vi "Get List Information.vi"(7 "App Instance":refnum<vi>, 8 "Tree DQMH Sel":string, 9 "DQMH Scan Info":T2, 11 "Tree Map":T4) -> (1 "Broadcast?":bool, 2 "Vi out":refnum<vi>, 3 "Module type":T1, 5 "DQMH Lib":refnum<vi>)   [LabVIEW 2019, in "Panther Dashboard.lvlib"]
uses:
  Panther Dashboard.lvlib
  <vilib>/National Instruments/Tree Map/Tree Map Data.ctl
  DQMH Modules Info--cluster.ctl
  Module type--enum.ctl
  Project References--cluster.ctl
  <vilib>/National Instruments/Tree Map/Tree Map.lvlib
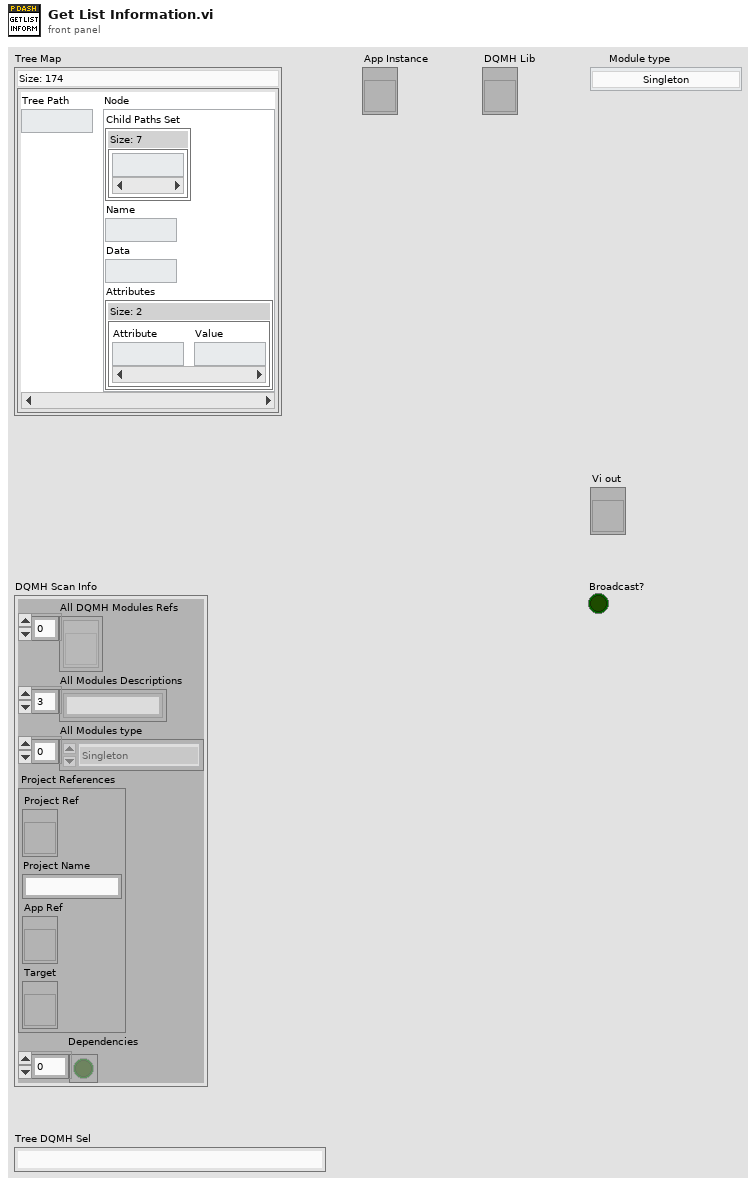
[diagram p1: front panel]
types:
  T1 = typedef "Panther Dashboard.lvlib/Module type--enum.ctl" = enum16{"Singleton", "Cloneable"}
  T2 = typedef "Panther Dashboard.lvlib/DQMH Modules Info--cluster.ctl" = cluster{"All DQMH Modules Refs":refnum<vi>[], "All Modules Descriptions":string[], "All Modules type":T1[], "Project References":T3, "Dependencies":bool[]}
  T3 = typedef "Panther Dashboard.lvlib/Project References--cluster.ctl" = cluster{"Project Ref":refnum<vi>, "Project Name":string, "App Ref":refnum<vi>, "Target":refnum<vi>}
  T4 = typedef "Tree Map.lvlib/Tree Map Data.ctl" = map{string, cluster{"Child Paths Set":set{string}, "Name":string, "Data":string, "Attributes":map{string, string}}}
  T5 = cluster{"Description":string, "VI Description":string}
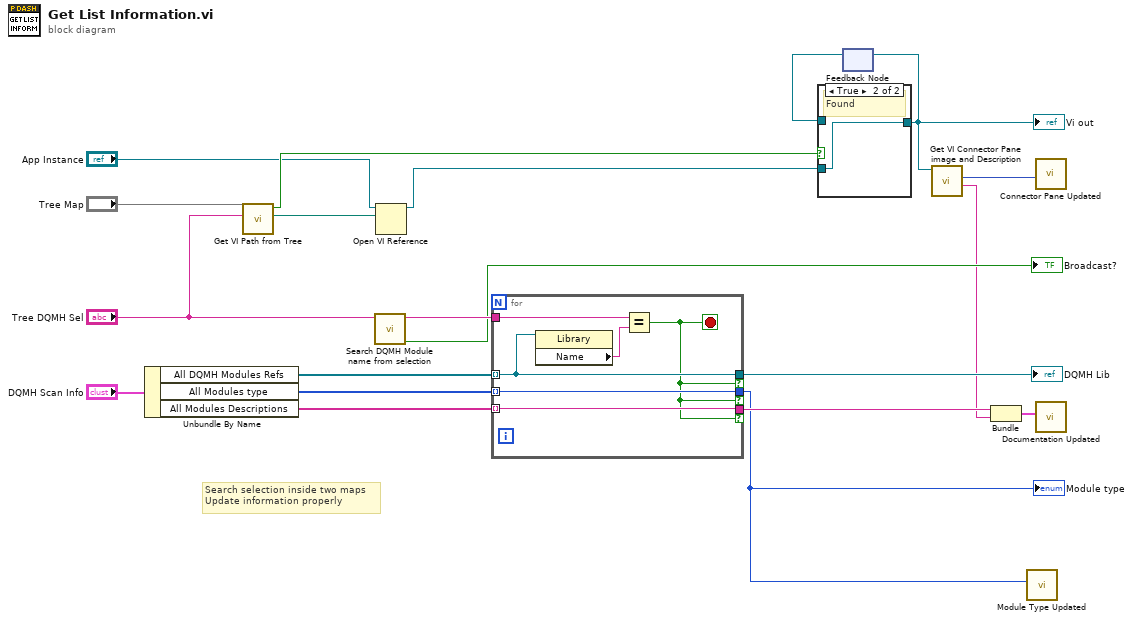
[diagram p0: block diagram]
diagram:
  # "Search selection inside two maps\nUpdate information properly"
  n1 = Unbundle By Name("DQMH Scan Info") -> ("All DQMH Modules Refs"=w19:refnum<vi>[], "All Modules type"=w18:T1[], "All Modules Descriptions"=w17:string[])
  n2 = call "Get VI Path from Tree.vi"("Tree Selection"="Tree DQMH Sel", "Tree Map"="Tree Map") -> ("path"=w10:path, "found?"=w7:bool)  [unwired: 8 in]
  n3 = call "Search DQMH Module name from selection.vi"("Search Module Name"="Tree DQMH Sel") -> ("Broadcast?"=→"Broadcast?":bool, "Module Name"=w16:string)  [unwired: 9 in]
  n4 = Open VI Reference(application reference (local)="App Instance", vi path=w10) -> (vi reference=w3:refnum<vi>)  [unwired: 4 in, 1 out]
  n5 = for {
    tunnel: w19 -> [w23] mode=indexing
    tunnel: w18 -> [w25] mode=indexing
    tunnel: w17 -> [w24] mode=indexing
    tunnel: w16 -> [w26]
    tunnel: [w23] -> w15 if=w21
    tunnel: [w25] -> w1 if=w21
    tunnel: [w24] -> w12 if=w21
    stop <- w21 stop-if-true
    n6 = property class="Library"(reference=w23) -> ("Name"=w22:string)  [unwired: 1 in, 2 out]
    n7 = Equal?(x=w26, y=w22) -> (x = y?=w21:bool)
  }
  "DQMH Lib" <- w15
  "Module type" <- w1
  n8 = feedback #1() -> (w14:refnum<vi>)  [unwired: 1 in]
  n9 = case shown="True" w7 {
    tunnel: [w27 w28] -> w2
    tunnel: w14 -> [w27 _]
    tunnel: w3 -> [_ w28]
    frame False {
      # "Not found"
    }
    frame True {
      # "Found"
    }
  }
  "Vi out" <- w2
  n10 = feedback-in #1(w2) -> ()
  n11 = call "Get VI Connector Pane image and Description.vi"("VI in"=w2) -> ("VI Description"=w5:string, "VI Connector Pane"=w4:picture)  [unwired: 7 in, 2 out]
  n12 = Bundle("Description"=w12, "VI Description"=w5) -> (w11:T5)  [unwired: 1 in]
  n13 = call "Module Type Updated.vi"("Module Type"=w1) -> ()  [unwired: 10 in, 1 out]
  n14 = call "Connector Pane Updated.vi"("Event Connector Pane"=w4) -> ()  [unwired: 10 in, 1 out]
  n15 = call "Documentation Updated.vi"("Documentation"=w11) -> ()  [unwired: 10 in, 1 out]
